vi "fftGetMax.vi"(9 "End Frequency (Hz)":i32=1385, 10 "Start Frequency (Hz)":i32=1355, 11 "Magnitudes":dbl[](array[numeric])) -> (3 "max value":dbl)   [LabVIEW 2011]
panel:
  out "subarray":dbl[](array[numeric])
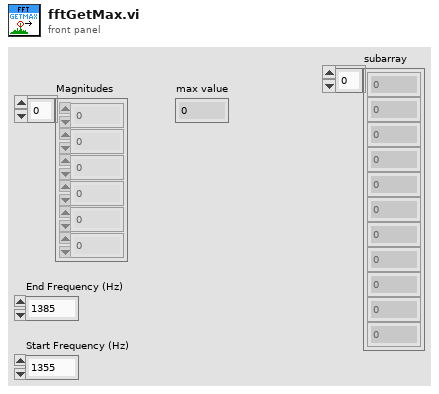
[diagram p1: front panel]
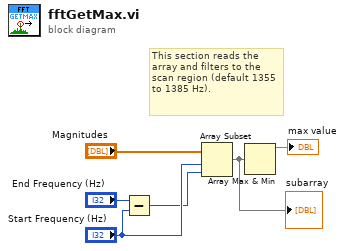
[diagram p0: block diagram]
diagram:
  # "This section reads the array and filters to the scan region (default 1355 to 1385 Hz)."
  n1 = Subtract(x="End Frequency (Hz)", y="Start Frequency (Hz)") -> (x-y=w2:i32)
  n2 = Array Subset(array="Magnitudes", index="Start Frequency (Hz)", length=w2) -> (w5:dbl[])
  "subarray" <- w5
  n3 = Array Max & Min(array=w5) -> (max value=→"max value":dbl)  [unwired: 3 out]
